vi "ReadFontStyle.vi"(7 "Fonts":T2[](array[typedef]), 8 "error in (no error)":errorcluster, 10 "Target Language":string) -> (0 "error out":errorcluster, 2 "Font Info":T1)   [LabVIEW 2019]
uses:
  Font Info -- Cluster.ctl
  Font -- Cluster.ctl
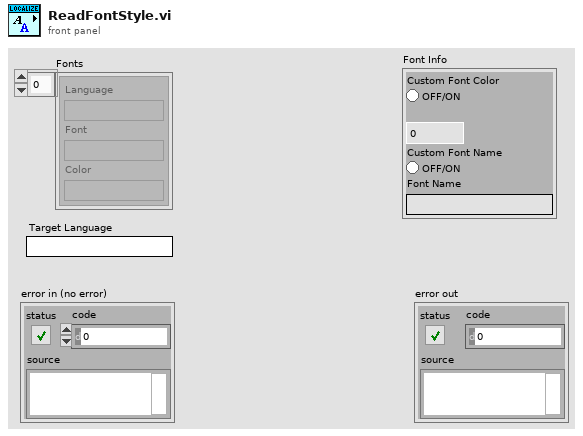
[diagram p1: front panel]
types:
  T1 = typedef "Font Info -- Cluster.ctl" = cluster{"Custom Font Color":bool, "Font Color":u32, "Custom Font Name":bool, "Font Name":string}
  T2 = typedef "Font -- Cluster.ctl" = cluster{"Language":string, "Font":string, "Color":string}
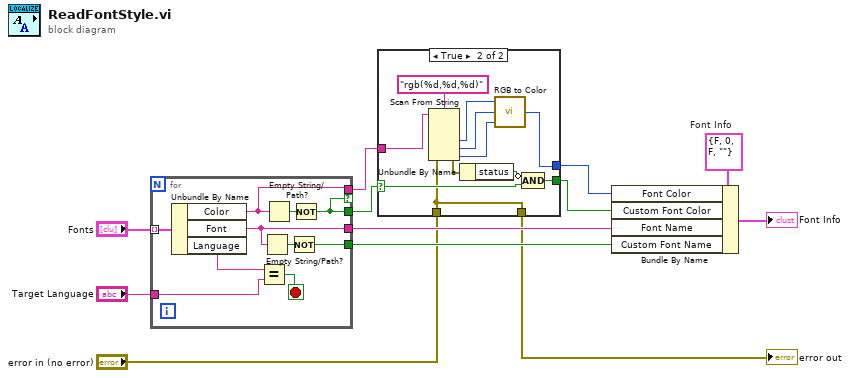
[diagram p0: block diagram]
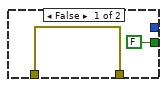
[diagram p2: hidden frame]
diagram:
  w12 = T1 {"Custom Font Color"=FALSE, "Font Color"=0, "Custom Font Name"=FALSE, "Font Name"=""}  # Font Info
  n1 = for {
    tunnel: "Fonts" -> [w22] mode=indexing
    tunnel: "Target Language" -> [w20]
    tunnel: [w13] -> w7
    tunnel: [w14] -> w8
    tunnel: [w16] -> w2
    tunnel: [w17] -> w6 if=w16
    stop <- w19 stop-if-true
    n2 = Unbundle By Name(w22) -> ("Color"=w17:string, "Font"=w14:string, "Language"=w21:string)
    n3 = Equal?(x=w21, y=w20) -> (x = y?=w19:bool)
    n4 = Empty String/Path?(string/path=w14) -> (empty?=w15:bool)
    n5 = Empty String/Path?(string/path=w17) -> (empty?=w18:bool)
    n6 = Not(x=w15) -> (.not. x?=w13:bool)
    n7 = Not(x=w18) -> (.not. x?=w16:bool)
  }
  n8 = case shown="True" w2 {
    selector: w2 -> [_ w27]
    tunnel: w6 -> [_ w35]
    tunnel: [_ w30] -> w5
    tunnel: "error in (no error)" -> [w24 w25]
    tunnel: [w24 w25] -> w3
    tunnel: [FALSE w26] -> w1
    frame False {
    }
    frame True {
      n9 = Scan From String(format string="rgb(%d,%d,%d)", input string=w35, error in=w25) -> (error out=w29:errorcluster, output 1=w33:i32, output 2=w32:i32, output 3=w31:i32)  [unwired: 4 in, 2 out]
      n10 = Unbundle By Name(w29) -> ("status"=w28:bool)
      n11 = call <vilib>:"RGB to Color.vi"("B"=w31, "G"=w32, "R"=w33) -> ("Color"=w30:u32)
      n12 = Compound Arithmetic op=AND(invert w28, w27) -> (w26:bool)
    }
  }
  "error out" <- w3
  n13 = Bundle By Name(cluster=w12, "Font Color"=w5, "Custom Font Color"=w1, "Font Name"=w8, "Custom Font Name"=w7) -> (→"Font Info":T1)
